vi "_MAIN - Dialog Demo.vi"() -> ()   [LabVIEW 2014]
uses:
  Flex UI (Parent)/Enum - Datum.ctl
  <vilib>/Utility/miscctls.llb/LVPositionTypeDef.ctl
  Flex UI Dialog/Flex UI Dialog.lvclass
  Flex UI (Parent)/Flex UI.lvclass
panel:
  in  "Position Settings":T3
  in  "Minimize":bool
  in  "Maximize":bool
  in  "Hide":bool
  in  "Show":bool
  in  "Launch":bool
  in  "Cleanup":bool
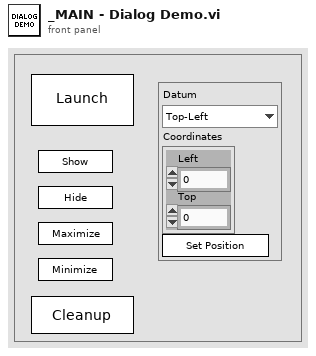
[diagram p1: front panel]
types:
  T1 = typedef "Flex UI.lvclass/Enum - Datum.ctl" = enum16{"Top-Left", "Top-Right", "Bottom-Left", "Bottom-Right", "Center"}
  T2 = typedef "LVPositionTypeDef.ctl" = cluster{"Left":i32, "Top":i32}
  T3 = cluster{"Datum":T1, "Coordinates":T2, "Set Position":bool}
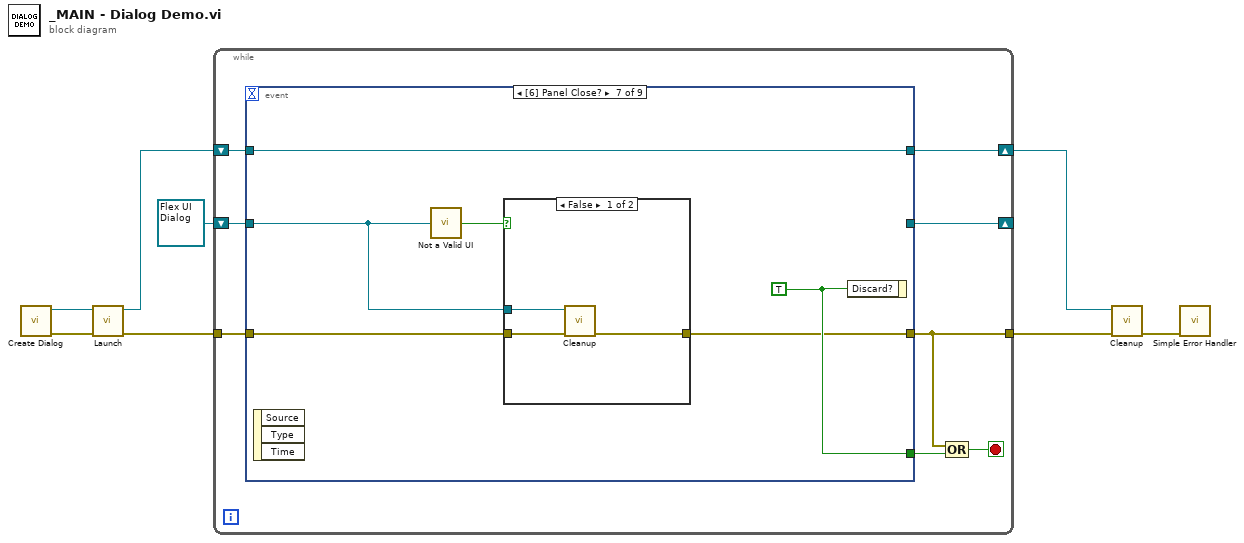
[diagram p0: block diagram]
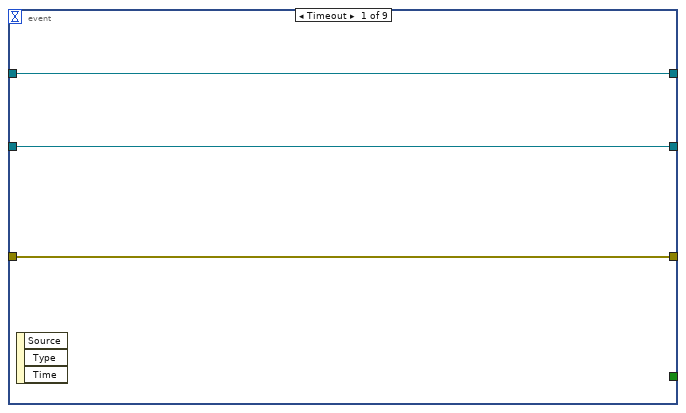
[diagram p2: hidden frame]
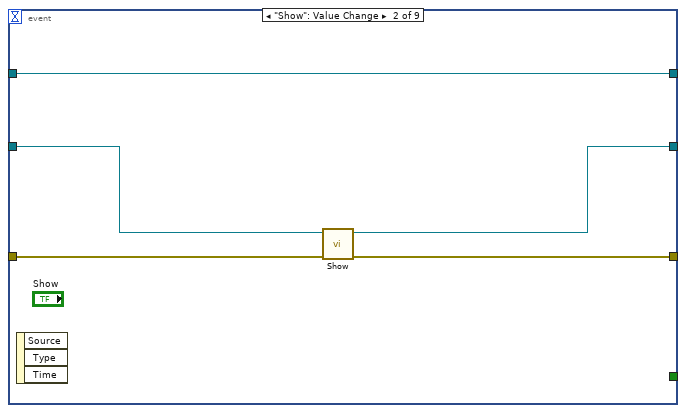
[diagram p3: hidden frame]
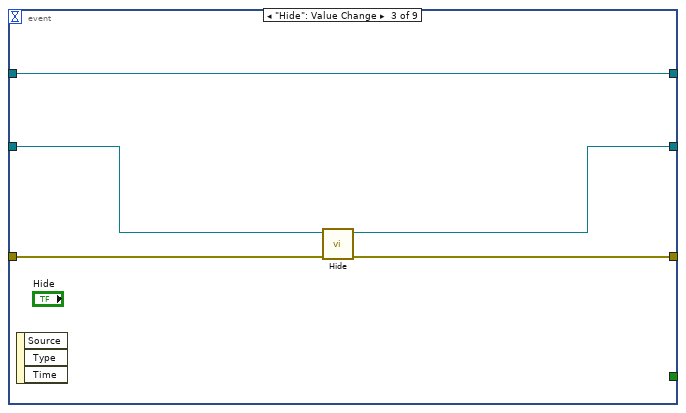
[diagram p4: hidden frame]
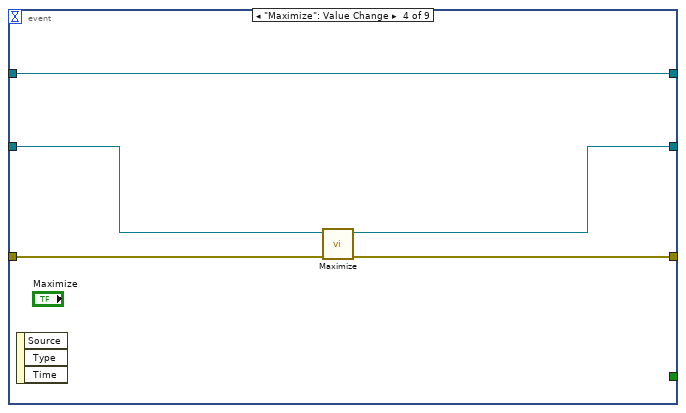
[diagram p5: hidden frame]
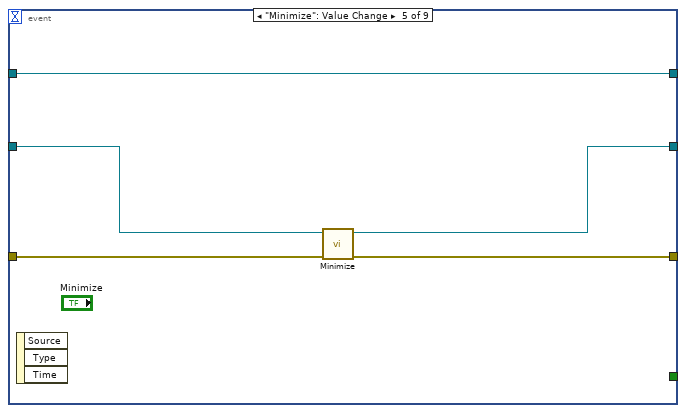
[diagram p6: hidden frame]
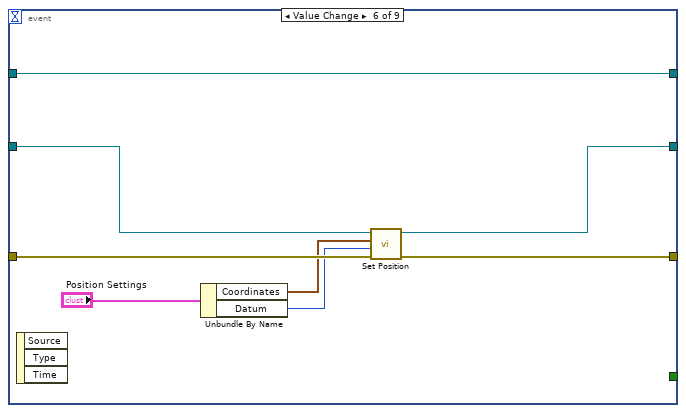
[diagram p7: hidden frame]
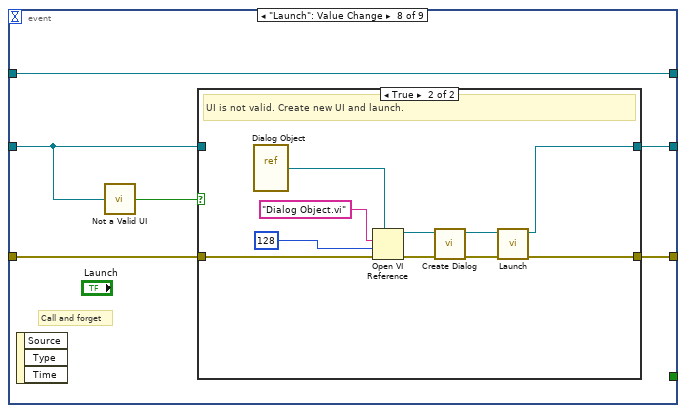
[diagram p9: hidden frame]
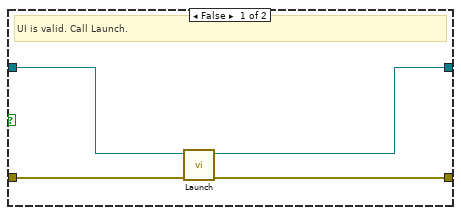
[diagram p10: hidden frame]
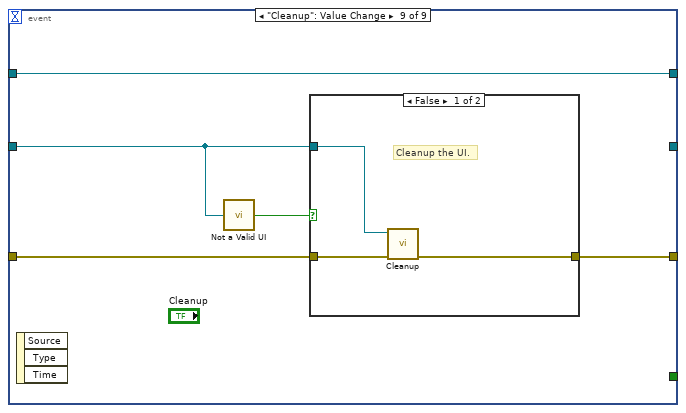
[diagram p11: hidden frame]
diagram:
  n1 = call "Create Dialog.vi"() -> ("error out"=w8:errorcluster, "Philips Dialog out"=w6:refnum<class "Flex UI Dialog.lvclass">)  [unwired: 10 in]
  n2 = call-dynamic "Launch.vi"("error in"=w8, "Philips Dialog in"=w6) -> ("error out"=w7:errorcluster, "Philips Dialog out"=w5:refnum<class "Flex UI Dialog.lvclass">)  [unwired: 8 in]
  n3 = while {
    tunnel: w7 -> [w14]
    shift-right: [w16] -> w4
    shift-left: w5 -> [w15]
    tunnel: [w11] -> w3
    shift-right: [w10] -> _
    shift-left: refnum<class "Flex UI Dialog.lvclass"> refnum ("Philips Dialog out") -> [w9]
    stop <- w12 stop-if-true
    n4 = event shown="[6] Panel Close?" {
      selector: _ -> [_ _ _ _ _ _ _ _ _]
      dyn-events: _ -> [_ _ _ _ _ _ _ _ _]
      timeout: _ -> [_ _ _ _ _ _ _ _ _]
      tunnel: [w19 w24 w29 w34 w39 w47 w53 w63 w82] -> w16
      tunnel: w15 -> [w19 w24 w29 w34 w39 w47 w53 w63 w82]
      tunnel: w14 -> [w18 w20 w25 w30 w35 w43 w52 w62 w80]
      tunnel: [w18 w21 w26 w31 w36 w44 w50 w61 w81] -> w11
      tunnel: [_ _ _ _ _ _ w51 _ _] -> w13
      tunnel: [w17 w23 w28 w33 w38 w46 _ w60 _] -> w10
      tunnel: w9 -> [w17 w22 w27 w32 w37 w45 w49 w59 w79]
      event Timeout {
        n5 = event-data() -> ()  [unwired: 1 in, 3 out]
      }
      event "Show": Value Change {
        n6 = event-data() -> ()  [unwired: 1 in, 3 out]
        n7 = call-dynamic "Show.vi"("error in"=w20, "Philips Dialog in"=w22) -> ("error out"=w21:errorcluster, "Philips Dialog out"=w23:refnum<class "Flex UI Dialog.lvclass">)  [unwired: 8 in]
      }
      event "Hide": Value Change {
        n8 = event-data() -> ()  [unwired: 1 in, 3 out]
        n9 = call-dynamic "Hide.vi"("error in"=w25, "Philips Dialog in"=w27) -> ("error out"=w26:errorcluster, "Philips Dialog out"=w28:refnum<class "Flex UI Dialog.lvclass">)  [unwired: 8 in]
      }
      event "Maximize": Value Change {
        n10 = event-data() -> ()  [unwired: 1 in, 3 out]
        n11 = call-dynamic "Maximize.vi"("error in"=w30, "Philips Dialog in"=w32) -> ("error out"=w31:errorcluster, "Philips Dialog out"=w33:refnum<class "Flex UI Dialog.lvclass">)  [unwired: 8 in]
      }
      event "Minimize": Value Change {
        n12 = event-data() -> ()  [unwired: 1 in, 3 out]
        n13 = call-dynamic "Minimize.vi"("error in"=w35, "Philips Dialog in"=w37) -> ("error out"=w36:errorcluster, "Philips Dialog out"=w38:refnum<class "Flex UI Dialog.lvclass">)  [unwired: 8 in]
      }
      event "Position Settings.Set Position": Value Change {
        n14 = event-data() -> ()  [unwired: 1 in, 3 out]
        n15 = Unbundle By Name("Position Settings") -> ("Coordinates"=w40:T2, "Datum"=w41:T1)
        n16 = call-dynamic "Set Position.vi"("error in"=w43, "Datum"=w41, "Target Coordinates"=w40, "Philips Dialog in"=w45) -> ("error out"=w44:errorcluster, "Philips Dialog out"=w46:refnum<class "Flex UI Dialog.lvclass">)  [unwired: 6 in]
      }
      event Panel Close? {
        w51 = TRUE ("Discard?")
        n17 = event-data() -> ()  [unwired: 1 in, 3 out]
        n18 = call "Not a Valid UI.vi"("Philips UI in"=w49) -> ("Not a Valid UI"=w48:bool)
        n19 = case shown="False" w48 {
          tunnel: w52 -> [w56 w57]
          tunnel: [w55 w57] -> w50
          tunnel: w49 -> [w54 _]
          frame False {
            n20 = call-dynamic "Cleanup.vi"("error in"=w56, "Philips Dialog in"=w54) -> ("error out"=w55:errorcluster)  [unwired: 9 in]
          }
          frame True {
          }
        }
        n21 = event-data("Discard?"=w51) -> ()  [unwired: 1 in, 1 out]
      }
      event "Launch": Value Change {
        # "Call and forget"
        n22 = event-data() -> ()  [unwired: 1 in, 3 out]
        n23 = call "Not a Valid UI.vi"("Philips UI in"=w59) -> ("Not a Valid UI"=w58:bool)
        n24 = case shown="True" w58 {
          tunnel: w62 -> [w67 w75]
          tunnel: [w66 w71] -> w61
          tunnel: [w64 w69] -> w60
          tunnel: w59 -> [w65 _]
          frame False {
            # "UI is valid. Call Launch."
            n25 = call-dynamic "Launch.vi"("error in"=w67, "Philips Dialog in"=w65) -> ("error out"=w66:errorcluster, "Philips Dialog out"=w64:refnum<class "Flex UI Dialog.lvclass">)  [unwired: 8 in]
          }
          frame True {
            # "UI is not valid. Create new UI and launch."
            n26 = vi-ref "Dialog Object.vi"() -> (w68:refnum<vi>)
            n27 = Open VI Reference(type specifier VI Refnum (for type only)=w68, vi path="Dialog Object.vi", options=128, error in (no error)=w75) -> (vi reference=w72:refnum<vi>, error out=w74:errorcluster)  [unwired: 2 in]
            n28 = call "Create Dialog.vi"("error in"=w74, "UI VI Reference (caller)"=w72) -> ("error out"=w73:errorcluster, "Philips Dialog out"=w70:refnum<class "Flex UI Dialog.lvclass">)  [unwired: 8 in]
            n29 = call-dynamic "Launch.vi"("error in"=w73, "Philips Dialog in"=w70) -> ("error out"=w71:errorcluster, "Philips Dialog out"=w69:refnum<class "Flex UI Dialog.lvclass">)  [unwired: 8 in]
          }
        }
      }
      event "Cleanup": Value Change {
        n30 = event-data() -> ()  [unwired: 1 in, 3 out]
        n31 = call "Not a Valid UI.vi"("Philips UI in"=w79) -> ("Not a Valid UI"=w78:bool)
        n32 = case shown="False" w78 {
          tunnel: [w85 w86] -> w81
          tunnel: w80 -> [w84 w86]
          tunnel: w79 -> [w83 _]
          frame False {
            # "Cleanup the UI."
            n33 = call-dynamic "Cleanup.vi"("error in"=w84, "Philips Dialog in"=w83) -> ("error out"=w85:errorcluster)  [unwired: 9 in]
          }
          frame True {
          }
        }
      }
    }
    n34 = Compound Arithmetic op=OR(w11, w13) -> (w12:bool)
  }
  n35 = call-dynamic "Cleanup.vi"("error in"=w3, "Philips Dialog in"=w4) -> ("error out"=w2:errorcluster)  [unwired: 9 in]
  n36 = call <vilib>:"Simple Error Handler.vi"("error in (no error)"=w2) -> ()  [unwired: 4 in, 5 out]
